vi "Split Text into Words.vi"(8 "error in (no error)":errorcluster) -> (0 "error out":errorcluster)   [LabVIEW 2021, in "Text-Based VI Icon Unit Tests.lvlib"]
doc: "Contains all the tests related to the function Split Text to Words"
uses:
  Text-Based VI Icon Unit Tests.lvlib
  <vilib>/addons/_JKI Toolkits/Caraya/classes/Assert/Assert Equal Value_Variant.vi
  <vilib>/LabVIEW Icon API/Set Text Icon/Text-Based VI Icon.lvlib
  <vilib>/addons/_JKI Toolkits/Caraya/classes/Test/Test.lvclass
  <vilib>/addons/_JKI Toolkits/Caraya/classes/Assert/Assert.lvclass
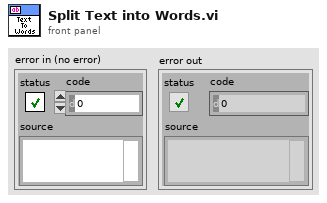
[diagram p1: front panel]
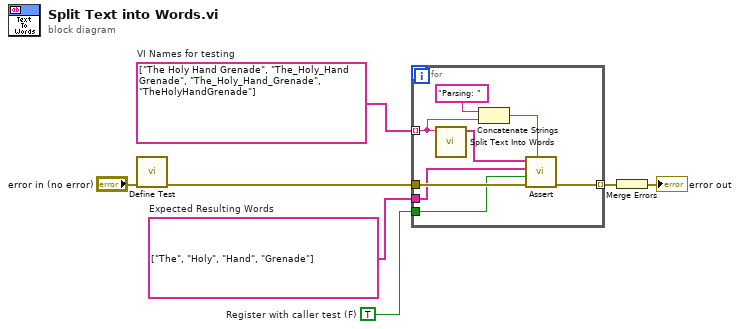
[diagram p0: block diagram]
diagram:
  w1 = TRUE  # Register with caller test (F)
  w5 = string[] ["The", "Holy", "Hand", "Grenade"]  # Expected Resulting Words
  w7 = string[] ["The Holy Hand Grenade", "The_Holy_Hand Grenade", "The_Holy_Hand_Grenade", "TheHolyHandGrenade"]  # VI Names for testing
  n1 = call <vilib>:"Define Test.vi"("error in (no error)"="error in (no error)") -> ("error out"=w6:errorcluster)  [unwired: 9 in, 1 out]
  n2 = for {
    tunnel: w7 -> [w11] mode=indexing
    tunnel: w6 -> [w15]
    tunnel: [w14] -> w4 mode=indexing
    tunnel: w5 -> [w13]
    tunnel: w1 -> [w8]
    n3 = call <vilib>:"Split Text Into Words.vi"("VI Name"=w11) -> ("Array"=w12:string[])  [unwired: 10 in]
    n4 = Concatenate Strings("Parsing: ", w11) -> (w9:string)
    n5 = call-poly <vilib>:"Assert.vi"("Label"=w9, "error in (no error)"=w15, "Register with caller test (F)"=w8, "Y"=w13, "X"=w12) -> ("error out"=w14:errorcluster)  [unwired: 5 in, 1 out]
  }
  n6 = Merge Errors(w4) -> (→"error out":errorcluster)
